vi "PLL -- data source -- V3 -- arydh.vi"(6 "set-get delay (msec)":i64, 7 "data source action":T2=enum."get", 9 "z  in (V)":cdb, 10 "Freq in (Hz)":dbl=40000.0 format="%#_13g", 11 "PLL data source":T1=enum."MFLI") -> (1 "z out (V)":cdb=0.00010527635459-2.9308681405e-05i, 2 "Freq out (Hz)":dbl=55115.2, 3 "PLL data source OUT":T1=enum."MFLI")   [LabVIEW 2019]
uses:
  publisher action.ctl
  PLL data source.ctl
  data source action.ctl
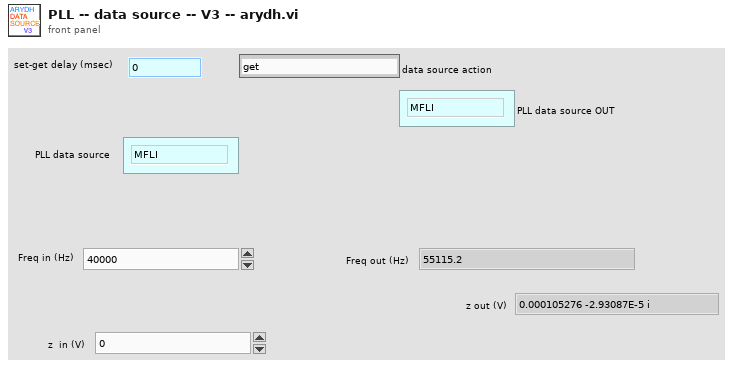
[diagram p1: front panel]
types:
  T1 = typedef "PLL data source.ctl" = enum16{"meta", "MFLI", "SRS865A", "arydh"}
  T2 = typedef "data source action.ctl" = enum16{"set", "get", "init", "set-and-get", "init source"}
  T3 = typedef "publisher action.ctl" = enum16{"set", "get", "init", "check"}
  T4 = typedef "MCL.lvlibp/MCL_DataRef.ctl" = refnum<vi>
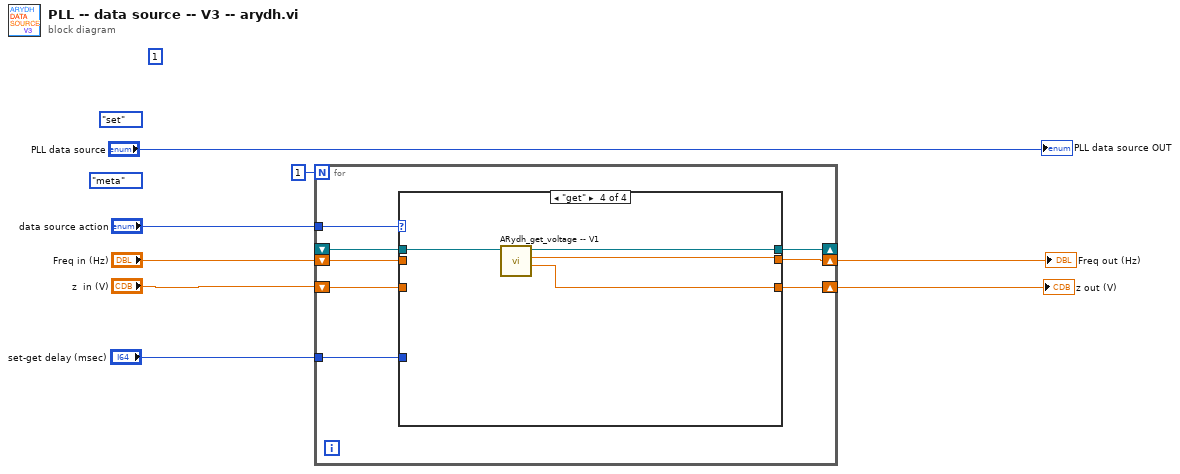
[diagram p0: block diagram]
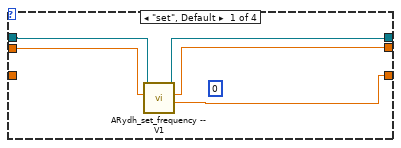
[diagram p2: hidden frame]
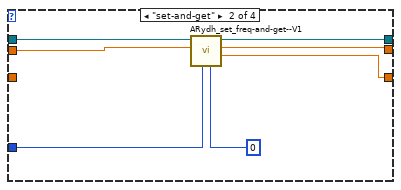
[diagram p3: hidden frame]
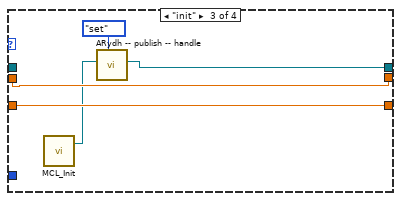
[diagram p4: hidden frame]
diagram:
  (unwired) 1
  (unwired) data_source_action."set" ("data source action")
  (unwired) PLL_data_source."meta" ("PLL data source")
  n1 = for {
    N: 1 -> [_]
    shift-right: [w16] -> _
    shift-left: _ -> [w15]
    shift-right: [w14] -> w7
    shift-left: "Freq in (Hz)" -> [w12]
    shift-right: [w13] -> w3
    shift-left: "z  in (V)" -> [w11]
    tunnel: "data source action" -> [w10]
    tunnel: "set-get delay (msec)" -> [w9]
    n2 = case shown="\"get\"" w10 {
      tunnel: [w20 w27 w31 w36] -> w16
      tunnel: w15 -> [w21 w28 _ w37]
      tunnel: [w18 w22 w32 w35] -> w14
      tunnel: [w17 w23 w33 w34] -> w13
      tunnel: w12 -> [w19 w26 w32 _]
      tunnel: w11 -> [_ _ w33 _]
      tunnel: w9 -> [_ w25 _ _]
      frame "set", Default {
        (unwired) u16 0 ("Oscillator (0)")
        n3 = call "ARydh_set_frequency -- V1.vi"("Freq in (Hz)"=w19, "MCL object"=w21) -> ("z out (V)"=w17:cdb, "Freq out (Hz)"=w18:dbl, "MCL object OUT"=w20:T4)  [unwired: 6 in, 1 out]
      }
      frame "set-and-get" {
        n4 = call "ARydh_set_freq-and-get--V1.vi"("Oscillator (0)"=u16 0, "delay-circle(msec)"=w25, "Freq in (Hz)"=w26, "MCL object"=w28) -> ("z out (V)"=w23:cdb, "Freq out (Hz)"=w22:dbl, "MCL object OUT"=w27:T4)  [unwired: 4 in, 1 out]
      }
      frame "init" {
        n5 = call "MCL_Init.vi"() -> ("MCL object"=w29:T4)  [unwired: 2 in, 1 out]
        n6 = call "ARydh -- publish -- handle.vi"("publisher action"=publisher_action."set", "MCL object"=w29) -> ("MCL object OUT"=w31:T4)  [unwired: 9 in]
      }
      frame "get" {
        n7 = call "ARydh_get_voltage -- V1.vi"("MCL object IN"=w37) -> ("z out (V)"=w34:cdb, "Freq out (Hz)"=w35:dbl, "MCL object OUT"=w36:T4)  [unwired: 7 in, 1 out]
      }
    }
  }
  "Freq out (Hz)" <- w7
  "z out (V)" <- w3
  "PLL data source OUT" <- "PLL data source"
